vi "App.OpenDatalogFlie.vi"(8 "error in (no error)":errorcluster, 11 "selected path":path) -> (0 "error out":errorcluster, 3 "Settings":T1)   [LabVIEW 2013, in "Simple Sequence Editor.lvlib"]
uses:
  Simple Sequence Editor.lvlib
  Types/Saved.Sequence.ctl
  Types/ChannelProperties.ctl
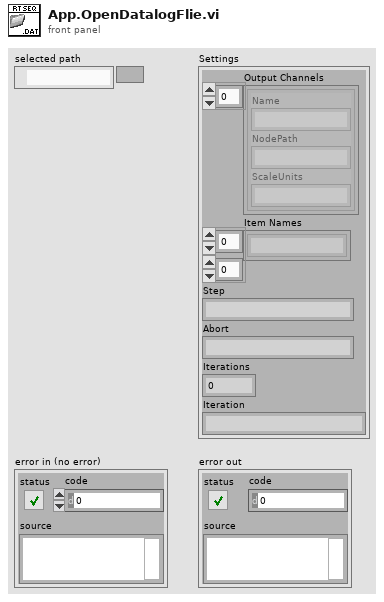
[diagram p1: front panel]
types:
  T1 = typedef "Simple Sequence Editor.lvlib/Saved.Sequence.ctl" = cluster{"Output Channels":T2[], "Item Names":string[][], "Step":string, "Abort":string, "Iterations":u32, "Iteration":string}
  T2 = typedef "Simple Sequence Editor.lvlib/ChannelProperties.ctl" = cluster{"Name":string, "NodePath":string, "ScaleUnits":string}
  T3 = enum16{"open", "replace", "create", "open or create", "replace or create", "replace or create with confirmation"}
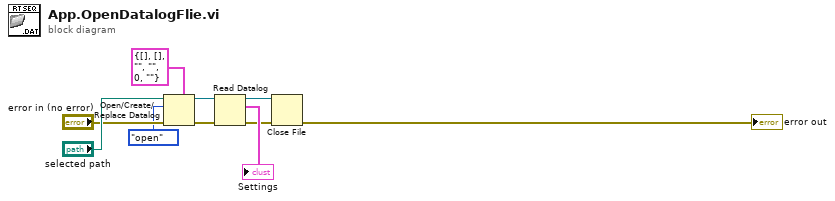
[diagram p0: block diagram]
diagram:
  n1 = Open/Create/Replace Datalog(5:T1 {"Output Channels"=[], "Item Names"=[], "Step"="", "Abort"="", "Iterations"=0, "Iteration"=""}, 8:"error in (no error)", 10:T3."open" ("operation (0:open)"), 11:"selected path") -> (0:w1:errorcluster, 3:w4:refnum<k1>)  [unwired: 2 in, 1 out]
  n2 = Read Datalog(4:w1, 7:w4) -> (0:w2:errorcluster, 2:→"Settings":T1, 3:w3:refnum<k1>)  [unwired: 1 in]
  n3 = Close File(refnum=w3, error in=w2) -> (error out=→"error out":errorcluster)  [unwired: 1 out]
